vi "fastFrame_config.vi"(8 "error in (no error)":errorcluster, 9 "Fast Frame":bool, 10 "fast frame count":i32, 11 "VISA resource name":refnum<visa-resource-name>) -> (0 "error out":errorcluster, 3 "VISA resource name out":refnum<visa-resource-name>)   [LabVIEW 2011]
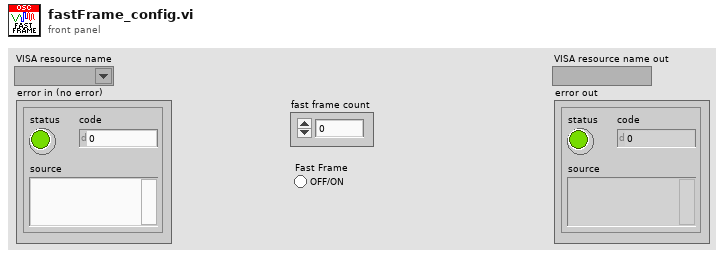
[diagram p1: front panel]
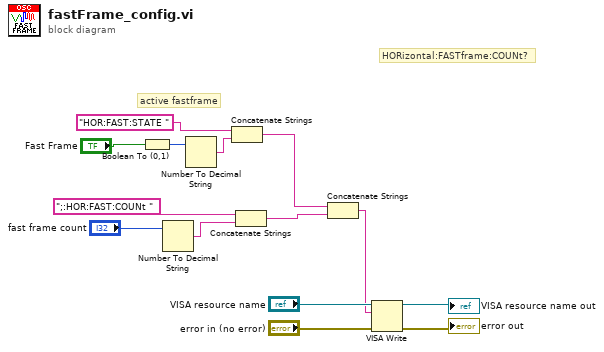
[diagram p0: block diagram]
diagram:
  # "HORizontal:FASTframe:COUNt?"
  # "active fastframe"
  n1 = Boolean To (0,1)(Boolean="Fast Frame") -> (0, 1=w13:i16)
  n2 = Number To Decimal String(number="fast frame count") -> (decimal integer string=w7:string)  [unwired: 1 in]
  n3 = Number To Decimal String(number=w13) -> (decimal integer string=w11:string)  [unwired: 1 in]
  n4 = Concatenate Strings("HOR:FAST:STATE ", w11) -> (w6:string)
  n5 = Concatenate Strings(";:HOR:FAST:COUNt ", w7) -> (w5:string)
  n6 = Concatenate Strings(w6, w5) -> (w4:string)
  n7 = VISA Write(VISA resource name="VISA resource name", write buffer=w4, error in (no error)="error in (no error)") -> (VISA resource name out=→"VISA resource name out":refnum<visa-resource-name>, error out=→"error out":errorcluster)  [unwired: 1 out]
